vi "Queue Driver.vi"(0 "Name":string, 5 "State":string, 7 "States[]":string[](array[string]), 11 "error in (no error)":errorcluster, 13 "Q Operations":T1) -> (4 "Dequeued State":string, 15 "error out":errorcluster)   [LabVIEW 2021, in "Queue Driver.lvlib"]
uses:
  Queue Driver.lvlib
  controls/Queue Operations.ctl
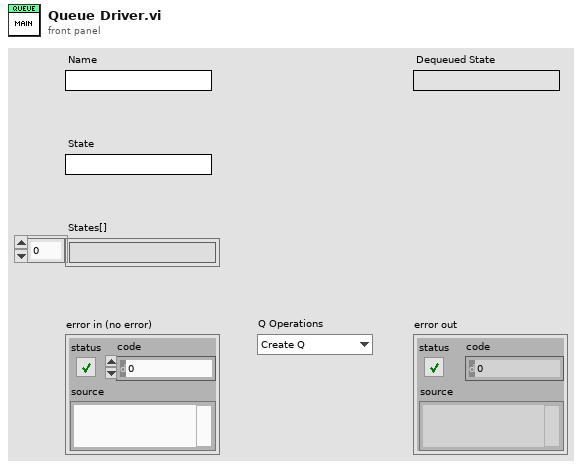
[diagram p1: front panel]
types:
  T1 = typedef "Queue Driver.lvlib/Queue Operations.ctl" = enum16{"Create Q", "Enqueue", "Enqueue N", "Dequeue", "Flush", "Release"}
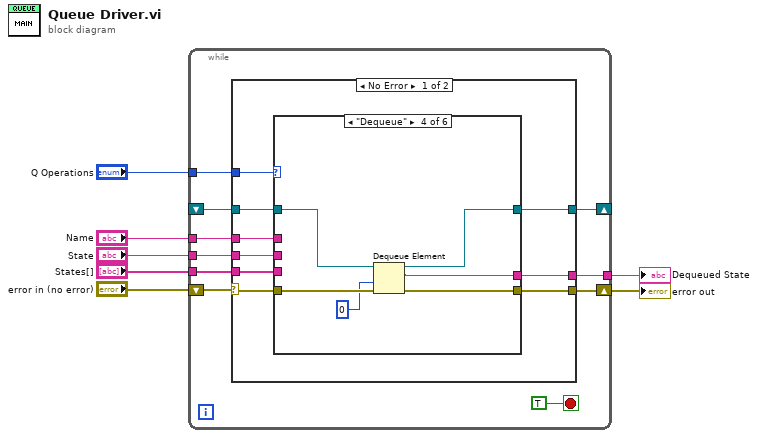
[diagram p0: block diagram]
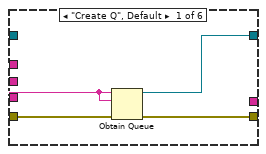
[diagram p2: hidden frame]
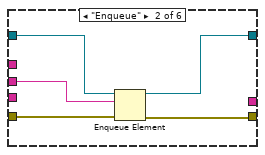
[diagram p3: hidden frame]
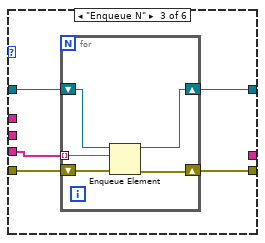
[diagram p4: hidden frame]
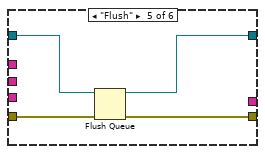
[diagram p5: hidden frame]
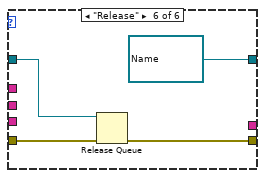
[diagram p6: hidden frame]
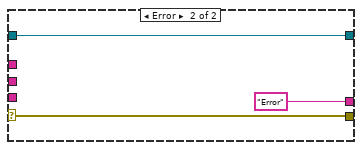
[diagram p7: hidden frame]
diagram:
  n1 = while {
    tunnel: "Q Operations" -> [w15]
    tunnel: "State" -> [w14]
    tunnel: "Name" -> [w13]
    tunnel: "States[]" -> [w12]
    shift-right: [w11] -> _
    shift-left: _ -> [w9]
    shift-right: [w10] -> w1
    shift-left: "error in (no error)" -> [w16]
    tunnel: [w8] -> w2
    stop <- TRUE stop-if-true
    n2 = case shown="No Error" w16 {
      selector: w16 -> [w23 w61]
      tunnel: w15 -> [w26 _]
      tunnel: w14 -> [w25 _]
      tunnel: w13 -> [w24 _]
      tunnel: w12 -> [w22 _]
      tunnel: [w21 w62] -> w11
      tunnel: [w20 w61] -> w10
      tunnel: w9 -> [w19 w62]
      tunnel: [w18 "Error" ("Name")] -> w8
      frame No Error {
        n3 = case shown="\"Dequeue\"" w26 {
          tunnel: w25 -> [_ w31 _ _ _ _]
          tunnel: w24 -> [w29 _ _ _ _ _]
          tunnel: w23 -> [w30 w35 w40 w51 w55 w58]
          tunnel: w22 -> [_ _ w36 _ _ _]
          tunnel: [w28 w33 w37 w48 w53 refnum<queue> refnum ("queue out")] -> w21
          tunnel: [w27 w34 w38 w50 w52 w56] -> w20
          tunnel: w19 -> [_ w32 w39 w49 w54 w59]
          tunnel: [_ _ _ w47 _ _] -> w18
          frame "Create Q", Default {
            n4 = Obtain Queue(name (unnamed)=w29, element data type=w29, error in (no error)=w30) -> (queue out=w28:refnum<queue>, error out=w27:errorcluster)  [unwired: 2 in, 1 out]
          }
          frame "Enqueue" {
            n5 = Enqueue Element(queue=w32, element=w31, error in (no error)=w35) -> (queue out=w33:refnum<queue>, error out=w34:errorcluster)  [unwired: 1 in, 1 out]
          }
          frame "Enqueue N" {
            n6 = for {
              shift-right: [w44] -> w38
              shift-left: w40 -> [w45]
              shift-right: [w42] -> w37
              shift-left: w39 -> [w43]
              tunnel: w36 -> [w41] mode=indexing
              n7 = Enqueue Element(queue=w43, element=w41, error in (no error)=w45) -> (queue out=w42:refnum<queue>, error out=w44:errorcluster)  [unwired: 1 in, 1 out]
            }
          }
          frame "Dequeue" {
            n8 = Dequeue Element(queue=w49, timeout in ms (-1)=0, error in (no error)=w51) -> (queue out=w48:refnum<queue>, element=w47:string, error out=w50:errorcluster)  [unwired: 1 out]
          }
          frame "Flush" {
            n9 = Flush Queue(queue=w54, error in (no error)=w55) -> (queue out=w53:refnum<queue>, error out=w52:errorcluster)  [unwired: 1 out]
          }
          frame "Release" {
            n10 = Release Queue(queue=w59, error in (no error)=w58) -> (error out=w56:errorcluster)  [unwired: 1 in, 2 out]
          }
        }
      }
      frame Error {
      }
    }
  }
  "error out" <- w1
  "Dequeued State" <- w2
